vi "HitrapGUI.StepMotorActivityNewDIM.vi"(0 "MotorName":string, 2 "Progress Slide Array":refnum<vi>[](array[refnum]), 3 "StartPosition":i32, 4 "StopPosition":i32, 5 "error in":errorcluster, 7 "Data":variant) -> (14 "Numeric":dbl, 16 "Finished?":bool, 19 "error out":errorcluster)   [LabVIEW 2014, in "HitrapGUI.lvlib"]
uses:
  HitrapGUI.lvlib
panel:
  in  "TR6DK1Ctl":T1 caption="TR6DK1" {"Progress Slide" scale=0.0..100.0; "Nom_Position" items=["Undefined", "Open", "Faraday Cup", "MCP"]}
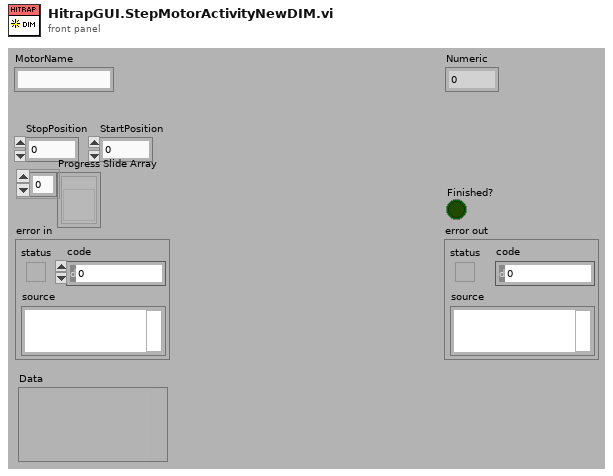
[diagram p1: front panel]
types:
  T1 = cluster{"Nom_Position":u8, "Progress Slide":u8, "TR6DK2Act":dbl, "TR6DK2Nom":dbl}
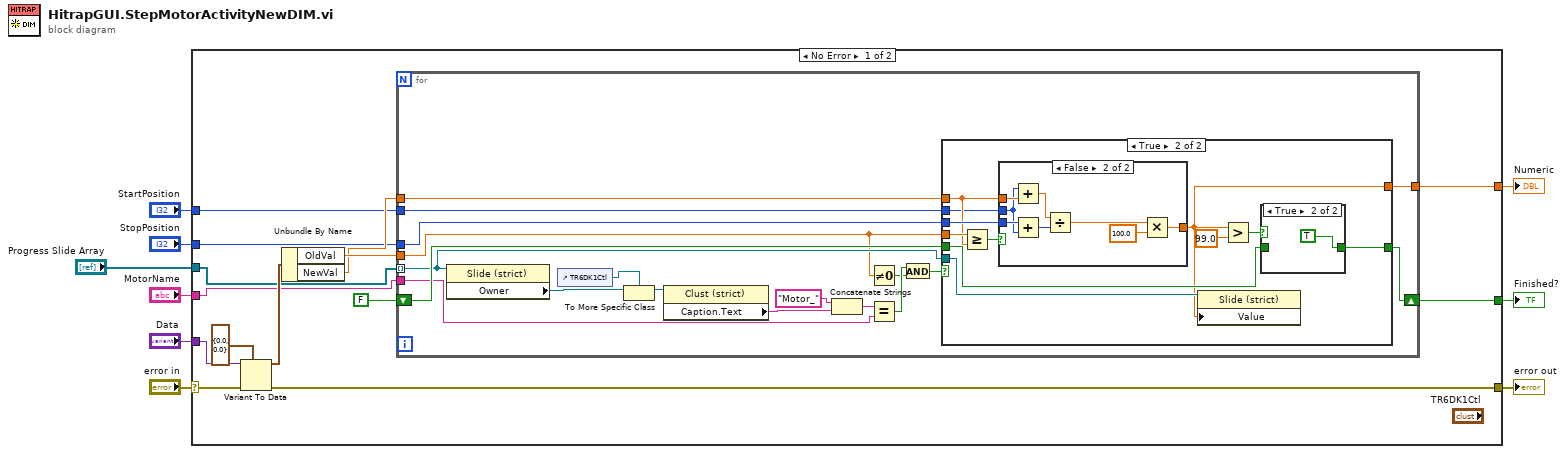
[diagram p0: block diagram]
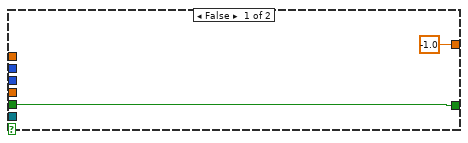
[diagram p2: hidden frame]
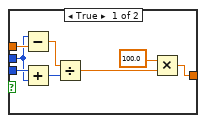
[diagram p4: hidden frame]
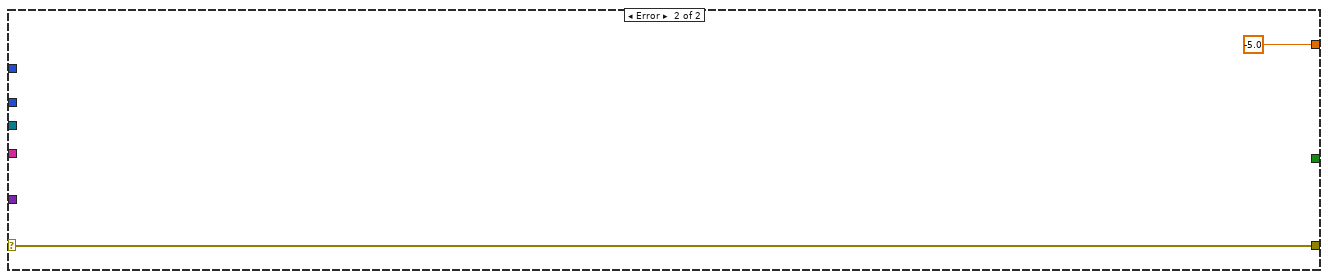
[diagram p5: hidden frame]
diagram:
  n1 = case shown="No Error" "error in" {
    selector: "error in" -> [w14 w74]
    tunnel: "StopPosition" -> [w19 _]
    tunnel: "StartPosition" -> [w18 _]
    tunnel: "Progress Slide Array" -> [w12 _]
    tunnel: [w16 _] -> w6
    tunnel: "Data" -> [w15 _]
    tunnel: [w13 w74] -> w3
    tunnel: "MotorName" -> [w11 _]
    tunnel: [w10 -5.0] -> w1
    frame No Error {
      n2 = Variant To Data(error in=w14, type=cluster{"OldVal":dbl, "NewVal":dbl} {"OldVal"=0.0, "NewVal"=0.0} ("output cluster"), Variant=w15) -> (data=w22:cluster{"OldVal":dbl, "NewVal":dbl}, error out=w13:errorcluster)
      n3 = Unbundle By Name(w22) -> ("OldVal"=w21:dbl, "NewVal"=w20:dbl)
      n4 = for {
        tunnel: w21 -> [w24]
        tunnel: w20 -> [w41]
        tunnel: w19 -> [w40]
        tunnel: w18 -> [w39]
        tunnel: w12 -> [w31] mode=indexing
        shift-right: [w37] -> w16
        shift-left: FALSE -> [w38]
        tunnel: w11 -> [w29]
        tunnel: [w28] -> w10
        n5 = property class="Slide (strict)"(reference=w31) -> ("Owner"=w32:refnum<vi>)  [unwired: 1 in, 2 out]
        n6 = control-ref of="TR6DK1Ctl"() -> (w33:refnum<vi>)
        n7 = To More Specific Class(target class=w33, reference=w32) -> (specific class reference=w34:refnum<vi>)  [unwired: 1 in, 1 out]
        n8 = property class="Clust (strict)"(reference=w34) -> ("Caption.Text"=w36:string)  [unwired: 1 in, 2 out]
        n9 = Concatenate Strings("Motor_" ("string"), w36) -> (w30:string)
        n10 = Not Equal To 0?(x=w24) -> (x != 0?=w25:bool)
        n11 = Equal?(x=w30, y=w29) -> (x = y?=w27:bool)
        n12 = And(x=w27, y=w25) -> (x .and. y?=w26:bool)
        n13 = case shown="True" w26 {
          tunnel: w31 -> [_ w54]
          tunnel: w24 -> [_ w53]
          tunnel: w41 -> [_ w50]
          tunnel: w40 -> [_ w51]
          tunnel: w39 -> [_ w49]
          tunnel: w38 -> [w43 w45]
          tunnel: [w43 w46] -> w37
          tunnel: [-1.0 w44] -> w28
          frame False {
          }
          frame True {
            n14 = Greater Or Equal?(x=w53, y=w50) -> (x >= y?=w52:bool)
            n15 = case shown="False" w52 {
              tunnel: w51 -> [w61 w69]
              tunnel: w50 -> [w64 w72]
              tunnel: w49 -> [w60 w68]
              tunnel: [w59 w67] -> w44
              frame True {
                n16 = Subtract(x=w60, y=w64) -> (x-y=w63:dbl)
                n17 = Add(x=w61, y=w60) -> (x+y=w62:i32)
                n18 = Divide(x=w63, y=w62) -> (x/y=w57:dbl)
                n19 = Multiply(x=100.0, y=w57) -> (x*y=w59:dbl)
              }
              frame False {
                n20 = Add(x=w68, y=w72) -> (x+y=w71:dbl)
                n21 = Add(x=w69, y=w68) -> (x+y=w70:i32)
                n22 = Divide(x=w71, y=w70) -> (x/y=w65:dbl)
                n23 = Multiply(x=w65, y=100.0) -> (x*y=w67:dbl)
              }
            }
            n24 = property class="Slide (strict)"(reference=w54, "Value"=w44) -> ()  [unwired: 1 in, 2 out]
            n25 = Greater?(x=w44, y=99.0) -> (0:w47:bool)
            n26 = case shown="True" w47 {
              tunnel: [w55 TRUE] -> w46
              tunnel: w45 -> [w55 _]
              frame False {
              }
              frame True {
              }
            }
          }
        }
      }
    }
    frame Error {
    }
  }
  "Finished?" <- w6
  "error out" <- w3
  "Numeric" <- w1
